vi "GetAccels.vi"() -> (3 "Initial Raw Accel":dbl[][](array[numeric]))   [LabVIEW 2013]
panel:
  in  "Initial Raw Accel 2":dbl[][](array[numeric])
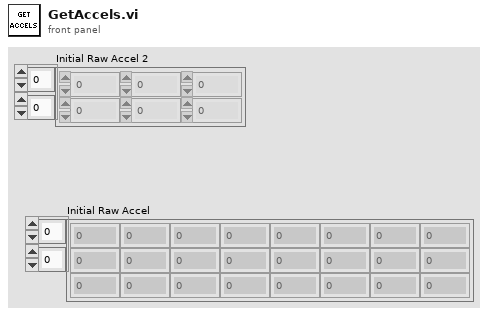
[diagram p1: front panel]
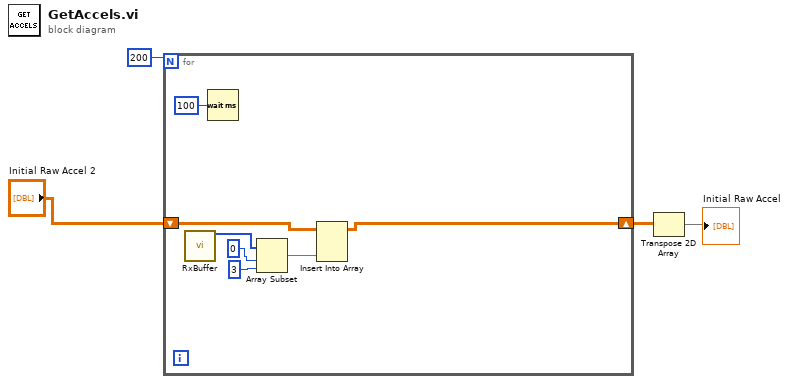
[diagram p0: block diagram]
diagram:
  n1 = for {
    N: 200 -> [_]
    shift-right: [w9] -> w2
    shift-left: "Initial Raw Accel 2" -> [w10]
    n2 = call "RxBuffer.vi"() -> ("RxData Out"=w6:u16[])  [unwired: 10 in, 9 out]
    n3 = Wait (ms)(milliseconds to wait=u32 100) -> ()  [unwired: 1 out]
    n4 = Array Subset(array=w6, index=0, length=3) -> (w5:u16[])
    n5 = Insert Into Array(array=w10, new element=w5) -> (w9:dbl[][])  [unwired: 2 in]
  }
  n6 = Transpose 2D Array(2D array=w2) -> (transposed array=→"Initial Raw Accel":dbl[][])
